vi "FTW-Actor-BeginShutdownSequence.vi"(1 "Jobs Prior to Shutdown Sequence":string, 3 "FTW Actor":refnum<class "FTW-Actor.lvclass">) -> (0 "FTW Actor out":refnum<class "FTW-Actor.lvclass">)   [LabVIEW 2014, in "FTW-Actor.lvclass"]
uses:
  FTW-Actor.lvclass
  Sequencer/FTW-Sequencer.lvclass
panel:
  # "Inputs"
  # "Outputs"
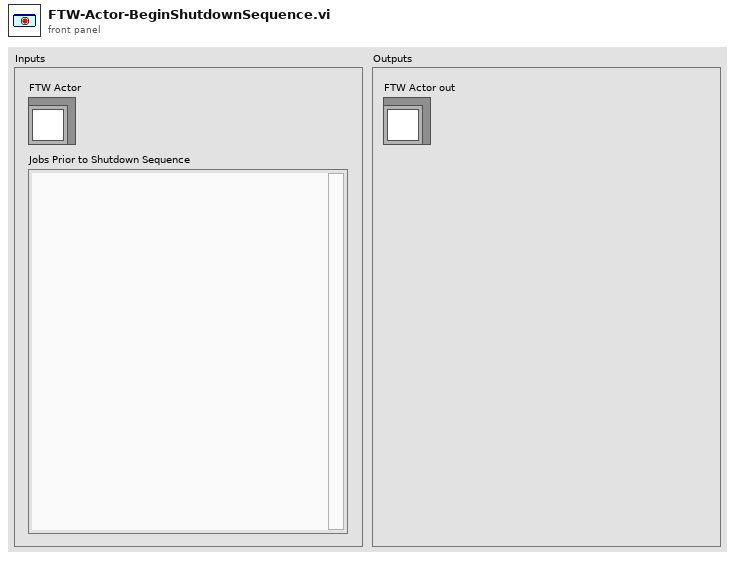
[diagram p1: front panel]
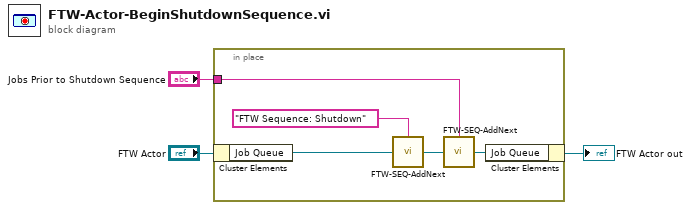
[diagram p0: block diagram]
diagram:
  n1 = in-place {
    in-place-border: "Jobs Prior to Shutdown Sequence" -> [w7]
    n2 = in-place-cluster #1("FTW Actor") -> ("Job Queue"=w6:refnum<class "FTW-Sequencer.lvclass">)
    n3 = call "FTW-SEQ-AddNext.vi"("Add Next in Sequence"="FTW Sequence: Shutdown", "Sequencer"=w6) -> ("Sequencer out"=w5:refnum<class "FTW-Sequencer.lvclass">)  [unwired: 2 in]
    n4 = call "FTW-SEQ-AddNext.vi"("Add Next in Sequence"=w7, "Sequencer"=w5) -> ("Sequencer out"=w8:refnum<class "FTW-Sequencer.lvclass">)  [unwired: 2 in]
    n5 = in-place-cluster #1("Job Queue"=w8) -> (→"FTW Actor out":refnum<class "FTW-Actor.lvclass">)
  }
